vi "Reanimate All.vi"(8 "Error In":errorcluster) -> (0 "Error Out":errorcluster)   [LabVIEW 2018, in "Tests.lvlib" / "Bookmark Manager.lvlib" / "Unit.lvlib"]
uses:
  Unit.lvlib
  <vilib>/addons/_JKI Toolkits/Caraya/classes/Test/Test.lvclass
  src/Bookmark Manager/Bookmark Manager.lvlib
  src/Toolkit/Toolkit.lvlib
  <vilib>/addons/_JKI Toolkits/Caraya/classes/Assert/Assert.lvclass
  Tests.lvlib
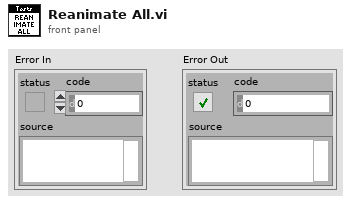
[diagram p1: front panel]
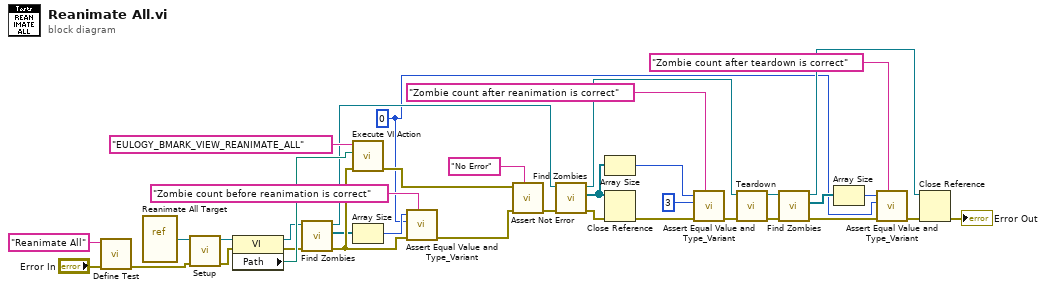
[diagram p0: block diagram]
diagram:
  w1 = 0 ("size(s)")
  n1 = call <vilib>:"Define Test.vi"("error in (no error)"="Error In", "Label (VI Title)"="Reanimate All") -> ("error out"=w35:errorcluster)  [unwired: 9 in]
  n2 = vi-ref "Reanimate All Target.vi"() -> (w34:refnum<vi>)
  n3 = call "Setup.vi"("Error In"=w35, "VI In"=w34) -> ("Error Out"=w32:errorcluster, "VI Out"=w31:refnum<vi>)  [unwired: 8 in]
  n4 = property on="Property Node" class="VI"(reference=w31, error in=w32) -> (reference out=w16:refnum<vi>, error out=w17:errorcluster, "Path"=w18:path)
  n5 = call "Find Zombies.vi"("Error In"=w17, "VI In"=w16) -> ("Error Out"=w14:errorcluster, "Graves"=w11:refnum<vi>[], "VI Out"=w15:refnum<vi>)  [unwired: 7 in]
  n6 = call "Execute VI Action.vi"("Error In"=w14, "VI"=w18, "Menu Tag"="EULOGY_BMARK_VIEW_REANIMATE_ALL") -> ("Error Out"=w26:errorcluster)  [unwired: 8 in]
  n7 = Array Size(array=w11) -> (size(s)=w10:i32)
  n8 = call <vilib>:"Assert Equal Value and Type_Variant.vi"("Label"="Zombie count before reanimation is correct", "error in (no error)"=w14, "Y"=w1, "X"=w10) -> ("error out"=w13:errorcluster)  [unwired: 7 in]
  n9 = call <vilib>:"Assert Not Error.vi"("Label"="No Error", "error in (no error)"=w13, "Not Error?"=w26) -> ("error out"=w25:errorcluster)  [unwired: 8 in]
  n10 = call "Find Zombies.vi"("Error In"=w25, "VI In"=w15) -> ("Error Out"=w28:errorcluster, "Graves"=w19:refnum<vi>[], "VI Out"=w23:refnum<vi>)  [unwired: 7 in]
  n11 = Array Size(array=w19) -> (size(s)=w30:i32)
  n12 = Close Reference(reference=w19, error in (no error)=w28) -> (error out=w20:errorcluster)
  n13 = call <vilib>:"Assert Equal Value and Type_Variant.vi"("Label"="Zombie count after reanimation is correct", "error in (no error)"=w20, "Y"=3 ("size(s)"), "X"=w30) -> ("error out"=w24:errorcluster)  [unwired: 7 in]
  n14 = call "Teardown.vi"("Error In"=w24, "VI In"=w23) -> ("Error Out"=w8:errorcluster, "VI Out"=w9:refnum<vi>)  [unwired: 8 in]
  n15 = call "Find Zombies.vi"("Error In"=w8, "VI In"=w9) -> ("Error Out"=w7:errorcluster, "Graves"=w3:refnum<vi>[], "VI Out"=w6:refnum<vi>)  [unwired: 7 in]
  n16 = Array Size(array=w3) -> (size(s)=w2:i32)
  n17 = call <vilib>:"Assert Equal Value and Type_Variant.vi"("Label"="Zombie count after teardown is correct", "error in (no error)"=w7, "Y"=w1, "X"=w2) -> ("error out"=w5:errorcluster)  [unwired: 7 in]
  n18 = Close Reference(reference=w6, error in (no error)=w5) -> (error out=→"Error Out":errorcluster)
